vi "RXRX 5785 No DDC Measure Phase Stability.vi"() -> (0 "error out":errorcluster)   [LabVIEW 2019]
uses:
  <vilib>/userDefined/Silver/nirio_resource_slv.ctl
  <instrlib>/FlexRIO/API/Host/v1/NI FlexRIO/API/Reference Clock Source.ctl
  Common/Original 5785 Example/Host/Upconversion Mode.ctl
  <instrlib>/niRFSG/niRFSG.llb/niRFSG Ref Clock Sources.ctl
  <vilib>/Analysis/1siggen.llb/Ramp Pattern by Delta.vi
  <instrlib>/FlexRIO/API/Host/v1/NI FlexRIO/API/Configure Reference Clock.vi
  <instrlib>/FlexRIO/API/Host/v1/NI FlexRIO/API/Get Property Reference - Fpga Small.vi
  <instrlib>/FlexRIO/API/Host/v1/NI FlexRIO/API/Configure Analog Start Trigger.vi
  <instrlib>/FlexRIO/API/Host/v1/NI FlexRIO/API/Configure Digital Edge Start Trigger.vi
  <instrlib>/FlexRIO/API/Host/v1/NI FlexRIO/API/Configure Immediate Start Trigger.vi
  <instrlib>/FlexRIO/API/Host/v1/NI FlexRIO/API/Read Stream 1D WDT.vi
  <vilib>/measure/matone.llb/Extract Single Tone Information N Chan.vi
  <vilib>/measure/maspectr.llb/FFT Power Spectrum and PSD for N Chan.vi
  <vilib>/FPGAPlugInAG/Dynamic/niLvFpga_Close_Dynamic.vi
  <vilib>/Utility/file.llb/Write Delimited Spreadsheet (DBL).vi
  <vilib>/rvi/interface/nirviCloseFPGA/nirviCloseFPGA.xnode
  <instrlib>/FlexRIO/API/Host/v1/NI FlexRIO API v1.lvlib
  <resource>/objmgr/niflexrioapiStream.rc
  <vilib>/measure/NI_MAPro.lvlib
  Common/Original 5785 Example/Host/GettingStarted_5785_Host.lvlib
  <vilib>/Analysis/NI_AALPro.lvlib
  <vilib>/Analysis/NI_AALBase.lvlib
panel:
  out "error out 2":errorcluster
  out "Results":T1(array[cluster])=[{"frequency (Hz)"=10000000.0, "mean skew"=-8.648150356036804e-11, "skew std dev"=2.4099744101288974e-11, "skew pk-pk"=7.257205272197028e-11, "skews"=[-7.634263492782065e-11, -5.206006966613256e-11, -7.567203753755032e-11, -1.2206425690719055e-10, -8.304777374940357e-11, -1.0474159284040468e-10, -9.611917176930304e-11, -4.9492204185220274e-11, -9.19555565839358e-11, -1.1331973743671892e-10]}, {"frequency (Hz)"=50000000.0, "mean skew"=-3.785636387258172e-12, "skew std dev"=7.66796131206532e-12, "skew pk-pk"=2.0450056958183634e-11, "skews"=[-1.4356702041335054e-11, -1.6858595580753508e-11, 3.9640356991197555e-13, 2.1898804487920657e-12, 3.591461377430126e-12, 5.627769488312176e-13, 2.0778793414142268e-12, -9.498878640875245e-13, -2.082260920467761e-12, -1.242731915231749e-11]}, {"frequency (Hz)"=100000000.0, "mean skew"=2.9756926970137243e-12, "skew std dev"=4.126438485430937e-12, "skew pk-pk"=1.3178656356672357e-11, "skews"=[-3.803864807523877e-12, 1.2229613162477112e-12, 3.353001868594509e-13, 6.147451569656316e-12, 3.467389040439413e-12, 9.37479154914848e-12, 3.130954906117878e-13, 5.3691066005407156e-12, 7.679194212684065e-12, -3.484981885268205e-13]}, {"frequency (Hz)"=150000000.0, "mean skew"=-3.1256285003637117e-12, "skew std dev"=2.50792505062644e-12, "skew pk-pk"=8.984925023293429e-12, "skews"=[-4.502762861812405e-12, -1.6045172273490561e-12, -2.9190171390647476e-12, -3.070990694678064e-13, -8.33215064320321e-12, -4.242400597204465e-12, -4.000839777166906e-12, 6.527743800902194e-13, -3.7005805394824356e-12, -2.2996915289763056e-12]}, {"frequency (Hz)"=200000000.0, "mean skew"=-8.350958023237677e-12, "skew std dev"=2.5975389756296594e-12, "skew pk-pk"=9.251979822405072e-12, "skews"=[-8.992508817543144e-12, -7.361526314260884e-12, -5.409418265633645e-12, -6.808722347470321e-12, -7.136097246425896e-12, -1.4661398088038717e-11, -1.0459370862648973e-11, -7.417267998914027e-12, -8.20329760295492e-12, -7.05997268848624e-12]}, {"frequency (Hz)"=250000000.0, "mean skew"=-6.229423609785982e-12, "skew std dev"=1.1181109842334413e-12, "skew pk-pk"=3.697563683201574e-12, "skews"=[-6.543472598258066e-12, -6.423877782336823e-12, -7.33916505767155e-12, -5.048427489200302e-12, -6.3111029457941555e-12, -6.605254632098134e-12, -6.962233060771497e-12, -3.95708736948471e-12, -5.448964109558302e-12, -7.654651052686284e-12]}, {"frequency (Hz)"=300000000.0, "mean skew"=-6.136089114075028e-12, "skew std dev"=9.42262857424596e-13, "skew pk-pk"=3.206385053636777e-12, "skews"=[-7.001117375279714e-12, -5.596228282724161e-12, -7.790788409887583e-12, -6.640956435014748e-12, -6.510029213872093e-12, -4.584403356250806e-12, -5.788671870420912e-12, -5.481861597872109e-12, -6.621852735719958e-12, -5.3449818637081885e-12]}, {"frequency (Hz)"=350000000.0, "mean skew"=-7.543098180047223e-12, "skew std dev"=3.8486735494540495e-13, "skew pk-pk"=1.2874637805991694e-12, "skews"=[-7.488662007824413e-12, -7.345064850347847e-12, -7.363173973336141e-12, -7.991225504656965e-12, -7.35831616172544e-12, -8.080201975318365e-12, -7.949579206730948e-12, -7.588239975011586e-12, -6.7927381947191955e-12, -7.473779950801325e-12]}, {"frequency (Hz)"=400000000.0, "mean skew"=-8.039336411333349e-12, "skew std dev"=7.425609882339821e-13, "skew pk-pk"=2.2738072930854095e-12, "skews"=[-7.656827769683663e-12, -9.457825738470782e-12, -7.679147937131138e-12, -7.995928800206408e-12, -8.83385230395903e-12, -7.54257226646767e-12, -7.31361750761873e-12, -7.184018445385372e-12, -7.962031171009181e-12, -8.767542173401512e-12]}, {"frequency (Hz)"=450000000.0, "mean skew"=-7.93200988579298e-12, "skew std dev"=7.97455496904726e-13, "skew pk-pk"=2.6238656725690157e-12, "skews"=[-7.898237136846618e-12, -8.55120393482239e-12, -8.79911402833156e-12, -7.812476697854857e-12, -7.693964239880247e-12, -6.482757646206027e-12, -8.3933125130091e-12, -9.106623318775042e-12, -7.260055680055343e-12, -7.322353662148608e-12]}, {"frequency (Hz)"=500000000.0, "mean skew"=-7.67982756908766e-12, "skew std dev"=6.672272359581462e-13, "skew pk-pk"=2.0371763701039724e-12, "skews"=[-8.507074422893644e-12, -7.0880582107488455e-12, -7.782804612094616e-12, -7.582126885479152e-12, -7.256810103118096e-12, -8.96121612129985e-12, -7.2605372159962215e-12, -7.281199578354681e-12, -6.924039751195878e-12, -8.154408789695609e-12]}, {"frequency (Hz)"=550000000.0, "mean skew"=-7.497637800191673e-12, "skew std dev"=7.103834430343908e-13, "skew pk-pk"=2.273387428636986e-12, "skews"=[-6.788566760330353e-12, -7.618981619747259e-12, -8.146972324445106e-12, -7.622320471598431e-12, -6.408580300349553e-12, -7.095092352672633e-12, -7.963135085088087e-12, -8.681967728986539e-12, -7.854698807254544e-12, -6.796062551444227e-12]}, {"frequency (Hz)"=600000000.0, "mean skew"=-6.656473926831814e-12, "skew std dev"=6.694881342261218e-13, "skew pk-pk"=1.9961300493555487e-12, "skews"=[-5.544977406952426e-12, -7.505826199727893e-12, -6.130703962050041e-12, -6.202863013065509e-12, -6.968667303110993e-12, -7.203039184312062e-12, -6.6392992458656125e-12, -6.0278794692841194e-12, -6.800376027641509e-12, -7.541107456307974e-12]}, {"frequency (Hz)"=650000000.0, "mean skew"=-6.170836312403341e-12, "skew std dev"=6.619061413781283e-13, "skew pk-pk"=2.2437727341724404e-12, "skews"=[-5.6761371841019825e-12, -6.355813112635683e-12, -5.813528117360099e-12, -5.8323315333927895e-12, -6.992345927519065e-12, -6.404883995266873e-12, -6.792134783464002e-12, -6.572966737937676e-12, -4.7485731933466245e-12, -6.5196485390086175e-12]}, {"frequency (Hz)"=700000000.0, "mean skew"=-6.189182831668323e-12, "skew std dev"=1.7157996931343636e-13, "skew pk-pk"=5.374178601958277e-13, "skews"=[-6.141615985942628e-12, -6.4858404095071854e-12, -6.233773633306086e-12, -6.2514132085703466e-12, -5.98652075251154e-12, -6.120870770642584e-12, -6.325272720314335e-12, -5.948422549311358e-12, -6.046719279911735e-12, -6.351379006665432e-12]}, {"frequency (Hz)"=750000000.0, "mean skew"=-6.5871572160487534e-12, "skew std dev"=4.41835545476434e-13, "skew pk-pk"=1.3482286990633495e-12, "skews"=[-6.408185337335485e-12, -6.6984014567953855e-12, -5.8037511563193215e-12, -5.956322167651966e-12, -6.385471028720583e-12, -7.009944685195322e-12, -6.796395481232521e-12, -6.839548682157055e-12, -6.821572309697221e-12, -7.151979855382671e-12]}, {"frequency (Hz)"=800000000.0, "mean skew"=-6.318415408299373e-12, "skew std dev"=5.360678898648873e-13, "skew pk-pk"=1.3845512042933417e-12, "skews"=[-6.991605843987897e-12, -6.471917002931961e-12, -5.868508226304447e-12, -6.587798178445769e-12, -5.6267669909771774e-12, -6.078767737351072e-12, -5.619707707506443e-12, -7.0042589117997844e-12, -6.851992861208232e-12, -6.082830622480952e-12]}, {"frequency (Hz)"=850000000.0, "mean skew"=-6.0180248346099665e-12, "skew std dev"=3.591713662163337e-13, "skew pk-pk"=1.1349470370084415e-12, "skews"=[-5.778738385130886e-12, -5.507329414754426e-12, -6.00610567960471e-12, -6.351181258112003e-12, -6.642276451762867e-12, -6.120739453272636e-12, -5.830550574804746e-12, -6.130742822105978e-12, -6.26599539616416e-12, -5.5465889103872445e-12]}, {"frequency (Hz)"=900000000.0, "mean skew"=-6.105366074378527e-12, "skew std dev"=2.6415729684293626e-13, "skew pk-pk"=9.150989335434855e-13, "skews"=[-6.100624138292147e-12, -6.176574316377945e-12, -6.247087188419655e-12, -6.696716487837525e-12, -5.835346835163569e-12, -5.994420432808338e-12, -6.201485877561482e-12, -5.78161755429404e-12, -5.8764077856967975e-12, -6.143380127333783e-12]}, {"frequency (Hz)"=950000000.0, "mean skew"=-6.431589636547766e-12, "skew std dev"=2.1126924807836585e-13, "skew pk-pk"=6.684732217835237e-13, "skews"=[-6.4527930268702555e-12, -6.67300399028584e-12, -6.020076613990734e-12, -6.561072065807103e-12, -6.250560131333176e-12, -6.440878292553848e-12, -6.404316276846632e-12, -6.580400983912426e-12, -6.244245148103377e-12, -6.6885498357742574e-12]}, {"frequency (Hz)"=1000000000.0, "mean skew"=-6.675839066411157e-12, "skew std dev"=3.266749368738765e-13, "skew pk-pk"=9.515417562958724e-13, "skews"=[-6.645668230188316e-12, -7.064422435097906e-12, -6.696684468644875e-12, -6.525650475721844e-12, -7.024648721850936e-12, -6.648717189793257e-12, -7.15475948867288e-12, -6.563526021551009e-12, -6.231095900213532e-12, -6.203217732377007e-12]}] {"frequency (Hz)" format="%#_6p"; "mean skew" format="%#_6p"; "skew std dev" format="%#_6p"; "skew pk-pk" format="%#_6p"; "skews" format="%#_6p"}
  out "Current Frequency Under Test":dbl=1000000000.0 format="%#_6p"
  in  "DUC Freq Shift (Hz)":dbl format="%#_4p"
  in  "DDC Freq Shift (Hz)":dbl format="%#_4p"
  in  "IQ Enabled":bool
  in  "DDC Enabled":bool
  in  "processing mode":T2=enum."None, Two Channels"
  out "AO num Samples":i32=160
  in  "waveform config":T3(array[cluster])=[{"Frequency (Hz)"=500000000.0, "Amplitude (V)"=0.2, "Phase (Deg)"=0.0}, {"Frequency (Hz)"=500000000.0, "Amplitude (V)"=0.20000000000000004, "Phase (Deg)"=0.0}] {"Phase (Deg)" format="%.2p"; "Amplitude (V)" format="%0.2p"; "Frequency (Hz)" format="%0.2p"}
  in  "reference clock source":T4 items=["Default", "Onboard", "PXI_Clk10", "External", "None", "Baseboard Reference"]
  in  "Update Waveform":bool caption="Download AO Waveforms"
  out "Sample Rate":dbl=3200000000.0 format="%#_6p"
  in  "ADC Interleaving Factor":i32=1 min=0 max=2 step=1
  in  "AI num samples":u64=1024 step=32
  in  "AI channels":string="AI0,AI1"
  out "Device Power":dbl(slide)=31.63 scale=-1.0..58.0 scale format="%#_3p"
  out "FPGA Temperature":dbl(slide)=48.0 scale=0.0..100.0 scale format="%#_3p"
  in  "Trigger Type":enum32{"Immediate", "Analog", "Digital"}(tab)
  in  "trigger channel":string="AI0"
  in  "rising edge?":bool=TRUE
  in  "level (V)":dbl format="%#_3p"
  in  "hysteresis (V)":dbl=0.01 format="%#_3p"
  in  "digital trigger source":string(combo)
  in  "stop":bool
  in  "Bitfile path":path=path "C:/Repos/bsherman-sandbox/CogRF/5785 Measurements/Common/Original 5785 Example/FPGA Bitfiles/PXIe_5785_KU060.lvbitx"
  in  "Waveform Tab Control":T5(tab)
  out "Waveform Graph":waveform(dbl)[](graph)
  out "FFT":cluster{"f0":dbl, "df":dbl, "magnitude":dbl[]}[](graph)=[{"f0"=0.0, "df"=3125000.0, "magnitude"=[-80.62408325882063, -85.86603200834055, -89.28274265648429, -98.83460657445366, -88.49970492095251, -87.20137991222401, -92.16186822162932, -88.63341970157178, -86.57322876142956, -81.27960143392245, -83.19897007752814, -101.03628298701321, -88.53320954191204, -97.6834958585654, -86.91305126564998, -83.50175897911802, -84.87430623302092, -85.85469273534017, -83.61501572265973, -92.60868045929556, -83.5487737269581, -95.57924716038043, -88.03819627141326, -87.8007109632868, -86.22942842860502, -93.88586113509106, -96.50099875515073, -101.76944809457721, -98.75888012640688, -93.50852632855973, -96.71449102628236, -95.26150214224074, -89.14320040806433, -88.19356759907032, -92.3717576813448, -86.26366547070903, -90.3640953616307, -97.0705350745329, -93.44506041606729, -83.45019580849757, -87.59607592004942, -93.04791056482202, -86.01950918085906, -91.76040050873144, -107.90090226718475, -95.54048362199053, -92.81892915821417, -90.49637721112424, -87.88362507998512, -91.35990300425655, -94.01965692391718, -97.15271627518251, -94.67940570840761, -87.43128756311114, -84.00666002576423, -84.8886135454118, -94.55974670647309, -81.32891176041906, -81.49826275796815, -83.61010416533553, -85.08969401858174, -86.2710734920104, -89.25397804822431, -84.35336325380959, -77.04679913737193, -79.44138684808263, -82.5521725429495, -85.07751517830293, -91.64743558874606, -94.29272208290016, -85.57125958138406, -82.63137130883501, -85.42117694615429, -89.7595979964928, -87.80930791115465, -97.05272987450931, -86.24684839017819, -92.7487208233722, -93.50722030363073, -89.71508571544445, -86.29678040775586, -88.43700064298288, -104.37542544129096, -100.6005180303963, -105.16052145956422, -88.35501528335524, -84.07762995516576, -89.11708736718252, -101.95791880747402, -101.11903982073274, -91.53564615323353, -89.68505577316223, -96.20655294838926, -88.24660836868955, -85.13464703714497, -87.09773569205302, -108.46658413769832, -93.5244048584424, -90.7762298779504, -88.8189672091992, -90.76265018556215, -89.52627637267476, -99.10427875864521, -93.88030078099446, -95.66794367896833, -94.86484286513401, -87.49037436640448, -84.25975439577809, -92.81025402846666, -102.14310591964161, -104.56438237821249, -88.79396016356577, -80.93202716361134, -79.69293470015937, -82.23898223787566, -86.86099114500065, -92.05216195480718, -97.2806041700401, -104.93908063005867, -102.00734373393934, -86.144191627308, -85.85716872484639, -106.95557108863434, -88.81397595160149, -82.08566536999571, -84.5526198841384, -102.54259872371915, -84.76938768891544, -80.18516684677365, -87.93966242225457, -92.35922797989657, -94.52158135899691, -97.27256222448466, -90.34462713703232, -92.95167044551575, -88.34061601459868, -86.6630051437812, -85.38073502586549, -84.66475771187625, -90.37681917853774, -87.47959315919672, -86.32257396570081, -89.88723621922546, -96.51239091072405, -88.4672651441393, -88.96065277473679, -103.27348718925435, -94.77179877524591, -86.58305070139056, -83.79206642170999, -87.7237680292307, -82.33915447429881, -82.34637165374383, -85.58842826936714, -111.1916469783211, -92.28860971952724, -96.14202725005923, -91.86358922692082, -102.5284899918548, -96.95228490572146, -89.21329891156824, -86.86723616442188, -80.55244748433157, -83.41476216896474, -89.58584951499597, -91.45404689819759, -88.2994355541738, -87.27531018981303, -89.11367011759623, -90.44968163374713, -91.89641030469662, -88.8665344705046, -88.17749850518986, -87.78788011530665, -91.09107551387129, -101.63801283891743, -97.00749373255141, -91.66041743463772, -92.42436859838949, -93.84542631249509, -89.14318161462872, -94.42514056615941, -91.82176529098876, -87.54179552722094, -96.1944119736967, -92.64102011012494, -91.80849877272553, -93.2509345517599, -97.46702201490821, -89.57764361479425, -87.10916067804374, -84.53756238317249, -84.29297673648031, -85.82470828754255, -87.32349940393595, -90.62969263730507, -90.65150086963344, -93.58592534321254, -91.98840539612276, -98.25886462346688, -97.87090010949308, -98.08113919441666, -87.48252593982764, -87.23427249557702, -86.32332994149834, -88.76977092083486, -87.17261795606083, -86.79648486397323, -93.87447143875792, -93.19702725712283, -84.65901927516336, -85.15545857076671, -88.17717673313815, -95.12508006828965, -93.37180286467299, -89.81410089936752, -91.70826662509879, -105.16237598121945, -92.28585826581272, -89.97750001073157, -98.03363246466297, -102.49644109820389, -103.58932772272428, -95.70054973964201, -89.38618304721759, -88.00523822460663, -86.7542519726739, -86.56284873200218, -83.56772658437664, -82.64158695029997, -87.02524508507662, -108.77054846509219, -96.75516700980094, -90.37920973563845, -91.55585427345716, -100.76580539709717, -91.00864385858671, -83.95403279844328, -95.00952027502932, -85.1002570310875, -88.37816798944269, -89.8964896357431, -88.7091119336639, -86.35067124920835, -90.46056069865298, -94.3078385527039, -84.62209100769655, -82.51278636544534, -91.32512707769337, -85.80555947690698, -83.97821250983651, -86.8839119686917, -88.14091163244555, -93.96127616450792, -93.32296993420931, -81.14652510994591, -78.40212557562388, -89.87926903352917, -92.80752789483628, -97.01446782079502, -101.53164569631124, -83.81585701201092, -83.69382877551594, -92.94115158287669, -96.16424112988054, -90.06888468381838, -92.29824324444479, -90.63701553273518, -90.17961203729266, -91.02942530299863, -96.96913821559535, -91.011027230546, -96.3033864841658, -90.16173642070942, -91.62035095729013, -87.45005679817208, -92.01984426943652, -95.37891685743662, -102.66339871574034, -95.89484652459541, -85.48121748128251, -85.33116010174561, -93.68398963167172, -90.89974327963404, -87.80333218256297, -94.8717784051056, -89.91162858797892, -96.61250811375906, -99.26768995204387, -102.92011070956511, -88.54120387485337, -88.1312594835668, -96.47343483348509, -90.46649283065834, -84.15249548962277, -85.11089955482512, -97.19528983826709, -87.65378120491647, -83.64022892119871, -87.93094137383859, -91.5197877641181, -87.56248194044835, -90.09334389471988, -91.48592654340929, -97.82606751390097, -89.50440806436391, -84.26741966919741, -90.07633885408111, -82.61109114310068, -85.10291510584915, -94.0483989349955, -93.3827423018114, -91.63560302024766, -87.26404452820424, -92.42859164266035, -98.0875260409756, -96.53327230929149, -92.46666683542617, -92.25287349594042, -31.083520536401082, -25.053441536208382, -31.05922543333303, -91.1340702535098, -83.44093015802356, -91.33797296859747, -90.28027862945106, -105.16688716473949, -88.86918433517062, -84.32057058677948, -83.28525952987539, -84.99268922610688, -87.1206168057242, -87.07908121653699, -83.63546629365999, -85.02724721384675, -94.37320165083986, -93.55506218441086, -87.69252631192332, -86.55648390510115, -89.02357821389153, -89.40635535541547, -94.2199312374972, -96.64164195211514, -84.9437137198135, -91.3839416256019, -86.91003312216395, -90.76758251849583, -98.52047130477942, -94.61726045894252, -91.20150587356052, -85.68547104146373, -86.65078830187248, -92.15709939981582, -91.00851065798452, -90.318359834728, -94.23742607884793, -88.3222513011706, -84.58042203608373, -92.36484549367484, -93.93372237660947, -90.3210552486612, -94.60720208299237, -94.06371815652774, -99.08416753286068, -91.5068696681547, -85.2986171937618, -85.81380335898382, -86.87960998531858, -89.70057378621851, -91.32272877938908, -88.6229441645375, -96.2094528930492, -98.1948045871535, -86.32017710554364, -82.9062419428689, -89.11849152793664, -88.81923930830689, -91.51711180429542, -88.23540249968536, -89.83463743883004, -95.41642246412425, -91.91956122823852, -92.80100754192841, -71.08890511957101, -65.67971161333253, -72.15132907853975, -92.25079517217141, -88.777280191169, -86.42306339406466, -88.59250499533044, -96.28666359438363, -107.02660438006626, -92.985964143596, -88.14043732618528, -87.51462348260569, -93.01530320218447, -86.27623092582397, -84.0157896049918, -83.50369116696727, -83.88175129246456, -86.20663415692674, -92.23320761694032, -92.08717301863116, -87.69561514787144, -100.47485887211477, -88.99000214555373, -91.20116400049159, -87.83008602254637, -84.42391938023489, -85.30665765205426, -88.4528647480578, -94.05190111800366, -86.27782068830611, -89.62029315886846, -87.80703876389089, -88.47526233702929, -89.6907447438686, -88.51856502206385, -102.04315460599096, -91.88897724249203, -98.57975862226054, -98.92272089239745, -93.8378680123593, -96.21218249758597, -106.81829498614434, -91.90504951784561, -89.18610324494207, -89.30156211559412, -103.94503562866618, -94.23602028790582, -92.82724657620983, -91.12854998451297, -89.52064178627612, -84.59009839283452, -82.40387164248722, -84.31816540589863, -86.25128458502704, -86.16473916831433, -91.01800245639724, -99.7236581399714, -97.9615894993939, -88.84460203374027, -89.904364864034, -91.5949187579583, -94.57023931182269, -89.40184353130165, -92.39613486661659, -90.94133334570691, -86.84032845552687, -89.5486004430567, -87.44960313388918, -90.73013656499151, -95.79677364532684, -91.48286321642176, -92.78729272209478, -86.91034246135419, -89.47605538332556, -87.26186051444219, -93.38284187770098, -88.1374271132297, -83.87513533087721, -93.5664817168523, -95.73881410854632, -96.86010215293203, -97.18644499670879, -94.20489845152736, -99.01566663750376, -93.26189262538972, -95.93025515033267, -91.5114728769568, -89.77761279736241, -101.19981254455168, -95.38229179293643, -87.11449185841309, -88.76678963090168, -91.3249073412343, -96.49438844661651, -90.37856717533815, -89.09822075924546, -89.31939400588264, -88.16558607784827, -88.16358039722442, -103.89477504410779, -92.06002375295917, -87.57101801286852, -85.5564608010288, -95.37316075308235, -89.65906559597066, -89.05243519614964, -85.01482725088141, -84.54359458482053, -93.82755904048577, -96.81378401682647, -93.81622520326978, -106.1760727709206, -86.6542435890689, -86.0481784823782, -85.75899913814617, -84.04631878480981, -84.20732443058316, -85.71273934992877, -96.66263897414544, -92.36829147291712, -88.55979759835441, -86.67853809486877, -84.79540824801303, -85.07986410147365, -88.45012557145039, -97.09569398216439, -84.80673445988637, -80.5083400679693, -79.81626397993568]}, ...(2 in all)] caption="Waveform Graph"
  out "detected frequencies":dbl[](array[numeric])=[1000003554.6699688, 1000002325.6067231] format="%_4p"
  out "AO Out":waveform(dbl)[](graph)=[{"t0"=timestamp(0 s since 1904-01-01), "dt"=3.125e-10, "Y"=[0.0, 0.16629392246050906, 0.1847759065022574, 0.03901806440322561, -0.1414213562373095, -0.19615705608064604, -0.07653668647301802, 0.11111404660392049, 0.2, 0.11111404660392035, -0.07653668647301787, -0.19615705608064607, -0.14142135623730956, 0.03901806440322578, 0.18477590650225734, 0.16629392246050892, 0.0, -0.16629392246050909, -0.18477590650225734, -0.03901806440322547, 0.14142135623730956, 0.196157056080646, 0.07653668647301785, -0.11111404660392055, -0.19999999999999996, -0.11111404660392023, 0.07653668647301798, 0.19615705608064604, 0.1414213562373094, -0.03901806440322589, -0.18477590650225728, -0.1662939224605088, 5.551115123125783e-17, 0.16629392246050909, 0.18477590650225723, 0.03901806440322533, -0.14142135623730945, -0.19615705608064585, -0.07653668647301788, 0.11111404660392057, 0.1999999999999999, 0.11111404660392012, -0.07653668647301798, -0.196157056080646, -0.14142135623730936, 0.03901806440322589, 0.18477590650225725, 0.16629392246050878, -2.7755575615628914e-17, -0.16629392246050906, -0.18477590650225725, -0.03901806440322536, 0.14142135623730942, 0.19615705608064593, 0.07653668647301794, -0.11111404660392066, -0.1999999999999999, -0.11111404660392014, 0.07653668647301792, 0.19615705608064604, 0.14142135623730945, -0.039018064403225916, -0.18477590650225728, -0.1662939224605088, 0.0, 0.16629392246050914, 0.18477590650225728, 0.03901806440322533, -0.14142135623730945, -0.19615705608064596, -0.07653668647301792, 0.11111404660392063, 0.1999999999999999, 0.11111404660392017, -0.07653668647301792, -0.1961570560806461, -0.14142135623730945, 0.039018064403226, 0.18477590650225728, 0.1662939224605088, 0.0, -0.1662939224605092, -0.18477590650225728, -0.039018064403225305, 0.14142135623730945, 0.196157056080646, 0.07653668647301792, -0.11111404660392071, -0.1999999999999999, -0.11111404660392012, 0.07653668647301792, 0.19615705608064615, 0.14142135623730945, -0.039018064403226055, -0.18477590650225728, -0.1662939224605088, 0.0, 0.16629392246050925, 0.18477590650225728, 0.039018064403225305, -0.14142135623730945, -0.19615705608064601, -0.07653668647301792, 0.11111404660392074, 0.1999999999999999, 0.11111404660392014, -0.07653668647301792, -0.1961570560806461, -0.14142135623730945, 0.03901806440322597, 0.18477590650225728, 0.1662939224605088, 0.0, -0.16629392246050914, -0.18477590650225728, -0.03901806440322539, 0.14142135623730945, 0.196157056080646, 0.07653668647301792, -0.1111140466039206, -0.1999999999999999, -0.11111404660392023, 0.07653668647301792, 0.19615705608064604, 0.14142135623730945, -0.03901806440322583, -0.18477590650225728, -0.16629392246050886, 0.0, 0.16629392246050909, 0.18477590650225728, 0.03901806440322539, -0.14142135623730945, -0.19615705608064593, -0.07653668647301792, 0.1111140466039206, 0.1999999999999999, 0.11111404660392019, -0.07653668647301792, -0.19615705608064607, -0.14142135623730945, 0.039018064403225944, 0.18477590650225728, 0.1662939224605088, 0.0, -0.16629392246050914, -0.18477590650225728, -0.03901806440322533, 0.14142135623730945, 0.19615705608064596, 0.07653668647301792, -0.11111404660392063, -0.1999999999999999, -0.11111404660392017, 0.07653668647301792, 0.1961570560806461, 0.14142135623730945, -0.039018064403226, -0.18477590650225728, -0.1662939224605088]}, {"t0"=timestamp(0 s since 1904-01-01), "dt"=3.125e-10, "Y"=[0.0, 0.16629392246050909, 0.1847759065022574, 0.03901806440322561, -0.1414213562373095, -0.19615705608064612, -0.07653668647301798, 0.11111404660392046, 0.20000000000000004, 0.11111404660392046, -0.076536686473018, -0.19615705608064612, -0.1414213562373095, 0.03901806440322561, 0.1847759065022574, 0.1662939224605091, 0.0, -0.166293922460509, -0.1847759065022574, -0.03901806440322575, 0.1414213562373095, 0.1961570560806461, 0.07653668647301802, -0.11111404660392044, -0.2, -0.11111404660392044, 0.07653668647301787, 0.1961570560806461, 0.14142135623730956, -0.03901806440322575, -0.18477590650225734, -0.16629392246050897, 0.0, 0.16629392246050903, 0.18477590650225734, 0.03901806440322558, -0.14142135623730956, -0.196157056080646, -0.07653668647301785, 0.11111404660392044, 0.19999999999999996, 0.11111404660392034, -0.07653668647301798, -0.196157056080646, -0.1414213562373094, 0.039018064403225666, 0.18477590650225728, 0.16629392246050895, -5.551115123125783e-17, -0.166293922460509, -0.18477590650225723, -0.039018064403225555, 0.14142135623730945, 0.19615705608064596, 0.07653668647301788, -0.11111404660392041, -0.1999999999999999, -0.11111404660392037, 0.07653668647301798, 0.196157056080646, 0.14142135623730936, -0.03901806440322561, -0.18477590650225725, -0.16629392246050897, 2.7755575615628914e-17, 0.16629392246050897, 0.18477590650225725, 0.03901806440322564, -0.14142135623730942, -0.19615705608064601, -0.07653668647301794, 0.11111404660392041, 0.1999999999999999, 0.11111404660392041, -0.07653668647301792, -0.19615705608064601, -0.14142135623730945, 0.03901806440322564, 0.18477590650225728, 0.16629392246050897, 0.0, -0.16629392246050897, -0.18477590650225728, -0.03901806440322564, 0.14142135623730945, 0.19615705608064601, 0.07653668647301792, -0.11111404660392041, -0.1999999999999999, -0.11111404660392041, 0.07653668647301792, 0.19615705608064601, 0.14142135623730945, -0.03901806440322564, -0.18477590650225728, -0.16629392246050897, 0.0, 0.16629392246050897, 0.18477590650225728, 0.03901806440322564, -0.14142135623730945, -0.19615705608064601, -0.07653668647301792, 0.11111404660392041, 0.1999999999999999, 0.11111404660392041, -0.07653668647301792, -0.19615705608064601, -0.14142135623730945, 0.03901806440322564, 0.18477590650225728, 0.16629392246050897, 0.0, -0.16629392246050897, -0.18477590650225728, -0.03901806440322564, 0.14142135623730945, 0.19615705608064601, 0.07653668647301792, -0.11111404660392041, -0.1999999999999999, -0.11111404660392041, 0.07653668647301792, 0.19615705608064601, 0.14142135623730945, -0.03901806440322564, -0.18477590650225728, -0.16629392246050897, 0.0, 0.16629392246050897, 0.18477590650225728, 0.03901806440322564, -0.14142135623730945, -0.19615705608064601, -0.07653668647301792, 0.11111404660392041, 0.1999999999999999, 0.11111404660392041, -0.07653668647301792, -0.19615705608064601, -0.14142135623730945, 0.03901806440322564, 0.18477590650225728, 0.16629392246050897, 0.0, -0.16629392246050897, -0.18477590650225728, -0.03901806440322564, 0.14142135623730945, 0.19615705608064601, 0.07653668647301792, -0.11111404660392041, -0.1999999999999999, -0.11111404660392041, 0.07653668647301792, 0.19615705608064601, 0.14142135623730945, -0.03901806440322564, -0.18477590650225728, -0.16629392246050897]}] caption="Waveform Graph"
  out "Limit (W)":dbl=58.0
  out "Power (W)":dbl=31.63
  out "Limit (C)":dbl=96.0
  out "Temp (C)":dbl=48.0 format="%#_4p"
  in  "RIO Device":T6="5785_00"
  # "Resource Configuration"
  # "Clocking configuration"
  # "Input Waveform Configuration"
  # "Device Monitoring"
  # "Output Waveform Configuration"
  # "Digital Upconverter Configuration"
  # "Frequency (Hz)"
  # "Amplitude (V)"
  # "Phase (Deg)"
  # "AO 0"
  # "AO 1"
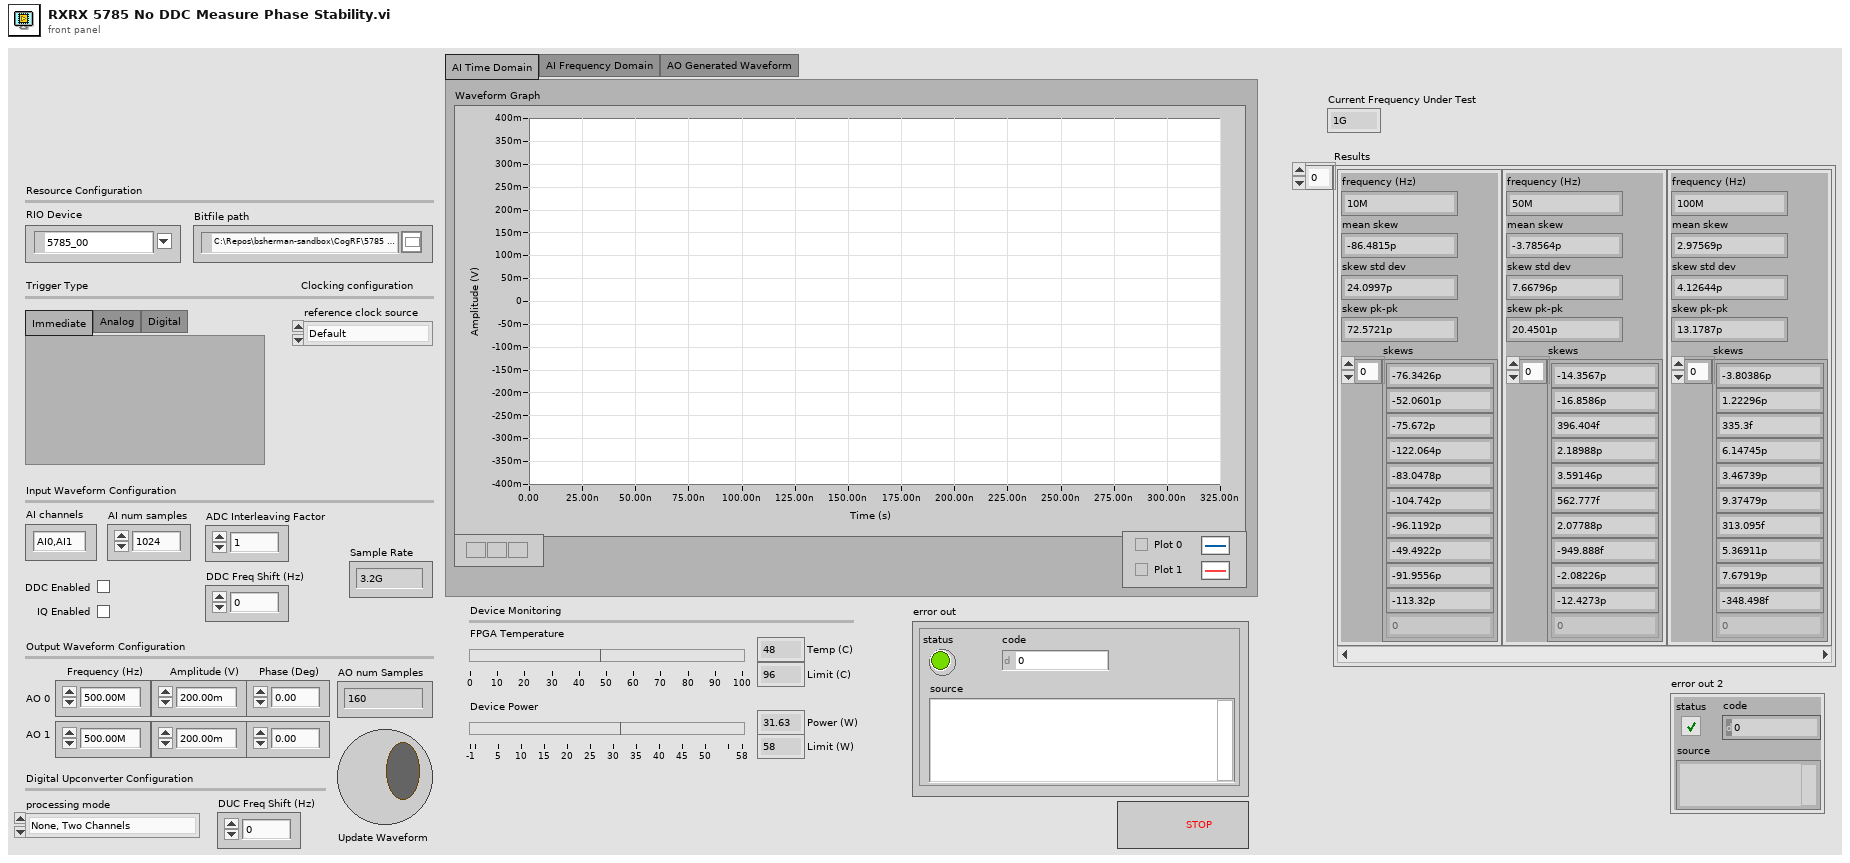
[diagram p1: front panel]
types:
  T1 = cluster{"frequency (Hz)":dbl, "mean skew":dbl, "skew std dev":dbl, "skew pk-pk":dbl, "skews":dbl[]}[]
  T2 = typedef "GettingStarted_5785_Host.lvlib/Upconversion Mode.ctl" = enum16{"None, One Channel", "None, Two Channels", "FPGA-only, One Channel", "DAC and FPGA, One Channel", "DAC-only, One Channel"}
  T3 = cluster{"Frequency (Hz)":dbl, "Amplitude (V)":dbl, "Phase (Deg)":dbl}[]
  T4 = typedef "NI FlexRIO API v1.lvlib/Reference Clock Source.ctl" = i32
  T5 = enum32{"AI Time Domain", "AI Frequency Domain", "AO Generated Waveform"}
  T6 = typedef "nirio_resource_slv.ctl" = tag
  T7 = typedef "niRFSG Ref Clock Sources.ctl" = string
  T8 = cluster{"frequency":dbl, "mean skew":dbl, "skew std dev":dbl, "skew pk-pk":dbl, "skews":dbl[]}
  T9 = cluster{"averaging mode":enum16{"No averaging", "Vector averaging", "RMS averaging", "Peak hold"}, "weighting mode":enum16{"Linear", "Exponential"}, "number of averages":u32}
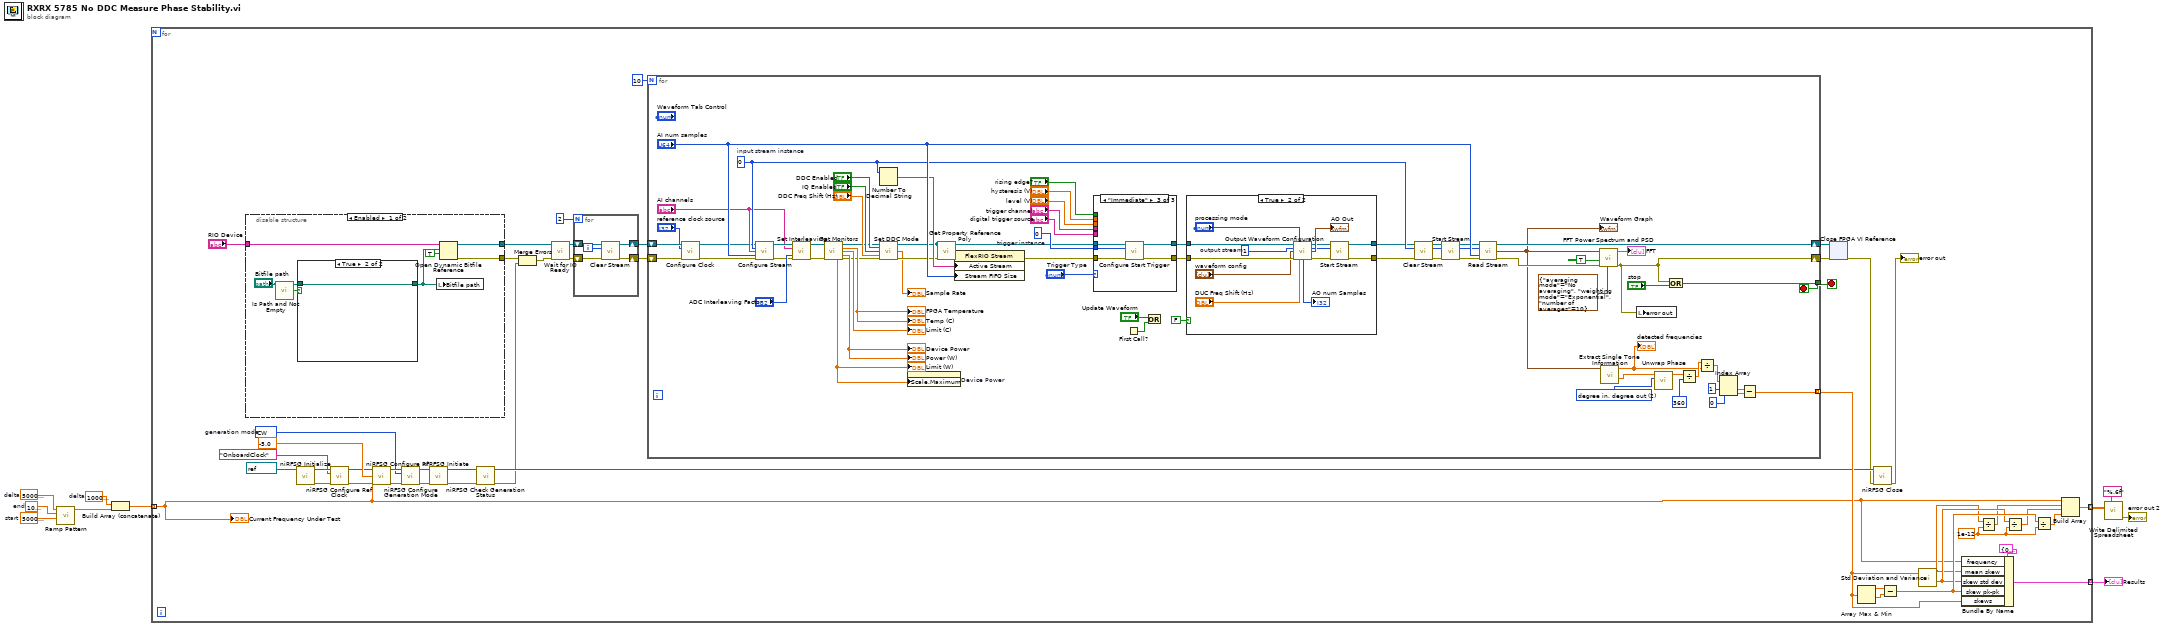
[diagram p0: block diagram]
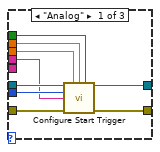
[diagram p3: hidden frame]
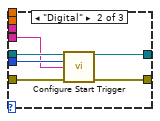
[diagram p4: hidden frame]
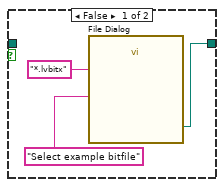
[diagram p5: hidden frame]
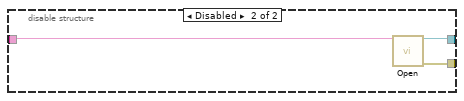
[diagram p6: hidden frame]
diagram:
  w6 = 10000000.0  # delta
  w8 = 50000000.0  # delta
  w9 = 1000000000.0  # end
  w10 = 50000000.0  # start
  n1 = call-poly <vilib>:"Ramp Pattern.vi"("start"=w10, "end"=w9, "delta"=w8) -> ("Ramp Pattern"=w7:dbl[])  [unwired: 6 in, 2 out]
  n2 = Build Array (concatenate)(w6, w7) -> (w2:dbl[])
  n3 = for {
    tunnel: [w33] -> w4 mode=indexing
    tunnel: [w32] -> w3 mode=indexing
    tunnel: w2 -> [w14] mode=indexing
    stop <- w44 stop-if-true
    w22 = 1000 items=["CW"=1000, "Arb Waveform"=1001, "Script"=1002]  # generation mode
    w34 = 1e-12 ("y")
    n4 = disable-structure shown="Enabled" {
      disable-tunnel: [w167 w174] -> w55
      disable-tunnel: [w166 w173] -> w54
      disable-tunnel: "RIO Device" -> [w165 w172]
      frame Enabled {
        n5 = call <vilib>:"Is Path and Not Empty.vi"("path"="Bitfile path") -> ("Is Path and Not Empty?"=w162:bool)  [unwired: 4 in]
        n6 = case shown="True" w162 {
          tunnel: "Bitfile path" -> [_ w171]
          tunnel: [w169 w171] -> w161
          frame False {
            n7 = call "File Dialog"("prompt"="Select example bitfile", "pattern (all files)"="*.lvbitx") -> ("selected path"=w169:path)  [unwired: 10 in, 3 out]
          }
          frame True {
          }
        }
        n8 = local write "Bitfile path"(w161) -> ()
        n9 = Open Dynamic Bitfile Reference(0:w165, 1:w161, 2:TRUE ("Run When Loaded")) -> (5:w166:refnum<k20>, 8:w167:errorcluster)  [unwired: 2 in]
      }
      frame Disabled {
        n10 = call <instrlib>:"Open.vi"("RIO Device"=w172) -> ("fpga interface out"=w173:refnum<k20>, "error out"=w174:errorcluster)  [unwired: 13 in]
      }
    }
    n11 = call <instrlib>:"niRFSG Initialize.vi"("resource name"=refnum<k15> "5652" ("Resource Name")) -> ("instrument handle"=w29:refnum<k15>, "error out"=w18:errorcluster)  [unwired: 13 in]
    n12 = call <instrlib>:"niRFSG Configure Ref Clock.vi"("instrument handle"=w29, "ref clock source"=T7 "OnboardClock" ("Clock Source"), "error in"=w18) -> ("instrument handle out"=w19:refnum<k15>, "error out"=w17:errorcluster)  [unwired: 11 in]
    n13 = call <instrlib>:"niRFSG Configure RF.vi"("instrument handle"=w19, "frequency (Hz)"=w14, "power level (dBm)"=-5.0 ("Power Level (dBm)"), "error in"=w17) -> ("instrument handle out"=w23:refnum<k15>, "error out"=w26:errorcluster)  [unwired: 10 in]
    n14 = call <instrlib>:"niRFSG Configure Generation Mode.vi"("instrument handle"=w23, "generation mode"=w22, "error in"=w26) -> ("instrument handle out"=w24:refnum<k15>, "error out"=w25:errorcluster)  [unwired: 11 in]
    n15 = call <instrlib>:"niRFSG Initiate.vi"("instrument handle"=w24, "error in"=w25) -> ("instrument handle out"=w28:refnum<k15>, "error out"=w15:errorcluster)  [unwired: 12 in]
    n16 = call <instrlib>:"niRFSG Check Generation Status.vi"("instrument handle"=w28, "error in"=w15) -> ("instrument handle out"=w27:refnum<k15>, "error out"=w13:errorcluster)  [unwired: 11 in, 1 out]
    n17 = Merge Errors(w55, w13) -> (w30:errorcluster)
    n18 = call <instrlib>:"Wait for IO Ready.vi"("fpga interface in"=w54, "error in"=w30) -> ("fpga interface out"=w50:refnum<k20>, "error out"=w49:errorcluster)  [unwired: 10 in, 2 out]
    n19 = for {
      N: 2 -> [_]
      shift-right: [w176] -> w47
      shift-left: w50 -> [w179]
      shift-right: [w177] -> w48
      shift-left: w49 -> [w178]
      i -> [w175]
      n20 = call <instrlib>:"Clear Stream.vi"("fpga interface in"=w179, "stream instance"=w175, "error in"=w178) -> ("fpga interface out"=w176:refnum<k20>, "error out"=w177:errorcluster)  [unwired: 10 in, 1 out]
    }
    n21 = for {
      N: 10 -> [_]
      shift-right: [w90] -> w51
      shift-left: w48 -> [w125]
      shift-right: [w123] -> w52
      shift-left: w47 -> [w124]
      tunnel: [w69] -> w44
      tunnel: [w56] -> w31 mode=indexing
      stop <- w69 stop-if-true
      w64 = 2 items=["radian in, radian out", "radian in, degree out", "degree in, degree out", "degree in, radian out"] ("phase unit")
      w114 = u32 0  # trigger instance
      w110 = u32 0  # input stream instance
      n22 = call-poly <instrlib>:"Configure Clock.vi"("fpga interface in"=w124, "reference clock source"="reference clock source", "error in"=w125) -> ("fpga interface out"=w92:refnum<k20>, "error out"=w118:errorcluster)  [unwired: 11 in]
      n23 = call <instrlib>:"Configure Stream.vi"("fpga interface in"=w92, "stream instance"=w110, "channels enabled"="AI channels", "num samples"="AI num samples", "error in"=w118) -> ("fpga interface out"=w108:refnum<k20>, "error out"=w106:errorcluster)  [unwired: 7 in, 2 out]
      n24 = call "Set Interleaving.vi"("fpga interface in"=w108, "AI channels enabled"="AI channels", "ADC Interleaving Factor"="ADC Interleaving Factor", "error in (no error)"=w106) -> ("fpga interface out"=w94:refnum<k20>, "error out"=w93:errorcluster)  [unwired: 10 in]
      n25 = call "Get Monitors.vi"("fpga interface in"=w94, "error in (no error)"=w93) -> ("fpga interface out"=w82:refnum<k20>, "FPGA Temperature (C)"=→"Temp (C)" →"FPGA Temperature":dbl, "Temperature Limit (C)"=→"Limit (C)":dbl, "Total Power (W)"=→"Power (W)" →"Device Power":dbl, "Power Limit (W)"=w100:dbl, "error out"=w81:errorcluster)  [unwired: 8 in]
      "Limit (W)" <- w100
      n26 = Number To Decimal String(number=w110) -> (decimal integer string=w116:string)  [unwired: 1 in]
      n27 = call "Set DDC Mode.vi"("fpga refnum"=w82, "DDC Enabled"="DDC Enabled", "IQ Enabled"="IQ Enabled", "DDC Frequency Shift (Hz)"="DDC Freq Shift (Hz)", "error in (no error)"=w81) -> ("fpga refnum out"=w83:refnum<k20>, "sample rate"=→"Sample Rate":dbl, "error out"=w84:errorcluster)  [unwired: 8 in]
      n28 = property on="Device Power" class="Slide (strict)"("Scale.Maximum"=w100) -> ()  [unwired: 2 in, 2 out]
      n29 = call-poly <instrlib>:"Get Property Reference Poly.vi"("error in (no error)"=w84, "fpga interface in"=w83) -> ("error out"=w105:errorcluster, "property reference"=w104:refnum<k20>)  [unwired: 4 in, 1 out]
      n30 = property class="FlexRIO Stream"(reference=w104, error in=w105, "Active Stream"=w116, "Stream FIFO Size"="AI num samples") -> (error out=w113:errorcluster)  [unwired: 1 out]
      n31 = case shown="\"Immediate\"" "Trigger Type" {
        tunnel: w83 -> [w149 w155 w160]
        tunnel: w113 -> [w148 w154 w159]
        tunnel: [w147 w153 w158] -> w112
        tunnel: [w146 w152 w157] -> w111
        tunnel: w114 -> [w145 w151 w156]
        tunnel: "trigger channel" -> [w144 _ _]
        tunnel: "level (V)" -> [w143 _ _]
        tunnel: "hysteresis (V)" -> [w142 _ _]
        tunnel: "rising edge?" -> [w141 _ _]
        tunnel: "digital trigger source" -> [_ w150 _]
        frame "Analog" {
          n32 = call-poly <instrlib>:"Configure Start Trigger.vi"("fpga interface in"=w149, "level"=w143, "hysteresis"=w142, "rising edge?"=w141, "trigger instance"=w145, "channel"=w144, "error in"=w148) -> ("fpga interface out"=w147:refnum<k20>, "error out"=w146:errorcluster)  [unwired: 6 in, 1 out]
        }
        frame "Digital" {
          n33 = call-poly <instrlib>:"Configure Start Trigger.vi"("fpga interface in"=w155, "trigger instance"=w151, "trigger source"=w150, "error in"=w154) -> ("fpga interface out"=w153:refnum<k20>, "error out"=w152:errorcluster)  [unwired: 9 in, 1 out]
        }
        frame "Immediate" {
          n34 = call-poly <instrlib>:"Configure Start Trigger.vi"("fpga interface in"=w160, "trigger instance"=w156, "error in"=w159) -> ("fpga interface out"=w158:refnum<k20>, "error out"=w157:errorcluster)  [unwired: 10 in, 1 out]
        }
      }
      n35 = First Call?() -> (First Call?: T/F=w78:bool)
      n36 = Or(x="Update Waveform", y=w78) -> ()  [unwired: 1 out]
      n37 = case shown="True" FALSE {
        tunnel: [w127 w140] -> w89
        tunnel: [w126 w139] -> w88
        tunnel: w112 -> [w127 w137]
        tunnel: w111 -> [w126 w136]
        frame False {
        }
        frame True {
          w133 = u32 1  # output stream
          n38 = call "Output Waveform Configuration.vi"("Refnum in"=w137, "processing mode"="processing mode", "output stream instance"=w133, "waveform config"="waveform config", "error in (no error)"=w136, "DUC Frequency Shift"="DUC Freq Shift (Hz)") -> ("Refnum out"=w134:refnum<k20>, "output stream instance out"=w132:u32, "waveforms out"=→"AO Out":waveform(dbl)[], "ao wfm samples"=→"AO num Samples":i32, "error out"=w135:errorcluster)  [unwired: 5 in]
          n39 = call <instrlib>:"Start Stream.vi"("fpga interface in"=w134, "stream instance"=w132, "error in"=w135) -> ("fpga interface out"=w140:refnum<k20>, "error out"=w139:errorcluster)  [unwired: 10 in, 1 out]
        }
      }
      n40 = call <instrlib>:"Clear Stream.vi"("fpga interface in"=w89, "stream instance"=w110, "error in"=w88) -> ("fpga interface out"=w76:refnum<k20>, "stream instance out"=w75:u32, "error out"=w74:errorcluster)  [unwired: 10 in]
      n41 = call <instrlib>:"Start Stream.vi"("fpga interface in"=w76, "stream instance"=w75, "error in"=w74) -> ("fpga interface out"=w72:refnum<k20>, "stream instance out"=w73:u32, "error out"=w71:errorcluster)  [unwired: 10 in]
      n42 = call-poly <instrlib>:"Read Stream.vi"("fpga interface in"=w72, "stream instance"=w73, "samples"="AI num samples", "error in"=w71) -> ("fpga interface out"=w123:refnum<k20>, "read data"=w58:waveform(dbl)[], "error out"=w96:errorcluster)  [unwired: 7 in, 2 out]
      "Waveform Graph" <- w58
      n43 = call-poly <vilib>:"FFT Power Spectrum and PSD.vi"("averaging parameters"=T9 {"averaging mode"=enum."No averaging", "weighting mode"=enum."Exponential", "number of averages"=10}, "error in (no error)"=w96, "dB On (F)"=TRUE, "time signals"=w58) -> ("error out"=w90:errorcluster, "Power Spectrum / PSD"=→"FFT":cluster{"f0":dbl, "df":dbl, "magnitude":dbl[]}[])  [unwired: 4 in, 2 out]
      n44 = call-poly <vilib>:"Extract Single Tone Information.vi"("time signals in"=w58) -> ("detected phases (deg)"=w63:dbl[], "detected frequencies"=w57:dbl[])  [unwired: 5 in, 4 out]
      "detected frequencies" <- w57
      n45 = local write "error out"(w90) -> ()
      n46 = call <vilib>:"Unwrap Phase.vi"("phase unit"=w64, "Phase"=w63) -> ("Unwrapped Phase"=w68:dbl[])  [unwired: 8 in, 1 out]
      n47 = Or(x=w90, y="stop") -> (x .or. y?=w69:bool)
      n48 = Divide(x=w68, y=360) -> (x/y=w67:dbl[])
      n49 = Divide(x=w67, y=w57) -> (x/y=w65:dbl[])
      n50 = Index Array(array=w65, index #1=1 ("index (row)"), index #2=0 ("index (row)")) -> (element #1=w60:dbl, element #2=w59:dbl)
      n51 = Subtract(x=w60, y=w59) -> (x-y=w56:dbl)
    }
    n52 = xnode "Close FPGA VI Reference"("FPGA VI Reference In"=w52, "error in"=w51) -> ("error out"=w12:errorcluster)
    n53 = Array Max & Min(array=w31) -> (max value=w37:dbl, min value=w36:dbl)  [unwired: 2 out]
    n54 = call <instrlib>:"niRFSG Close.vi"("instrument handle"=w27, "error in"=w12) -> ("error out"=→"error out":errorcluster)  [unwired: 13 in]
    n55 = Subtract(x=w37, y=w36) -> (x-y=w42:dbl)
    n56 = call <vilib>:"Std Deviation and Variance.vi"("X"=w31) -> ("mean"=w38:dbl, "standard deviation"=w40:dbl)  [unwired: 1 in, 1 out]
    n57 = Bundle By Name(cluster=T8 {"frequency"=0.0, "mean skew"=0.0, "skew std dev"=0.0, "skew pk-pk"=0.0, "skews"=[]}, "frequency"=w14, "mean skew"=w38, "skew std dev"=w40, "skew pk-pk"=w42, "skews"=w31) -> (w32:T8)
    n58 = Divide(x=w38, y=w34) -> (x/y=w39:dbl)
    n59 = Divide(x=w40, y=w34) -> (x/y=w41:dbl)
    n60 = Divide(x=w42, y=w34) -> (x/y=w43:dbl)
    n61 = Build Array(w14, w39, w41, w43) -> (w33:dbl[])
    "Current Frequency Under Test" <- w14
  }
  "Results" <- w3
  n62 = call-poly <vilib>:"Write Delimited Spreadsheet.vi"("format (%.3f)"="%.6f", "2D data"=w4) -> ("error out"=→"error out 2":errorcluster)  [unwired: 12 in, 1 out]
